vi "Set UI Busy State.vi"(7 "Defer Panel Updates":bool, 8 "error in (no error)":errorcluster, 11 "VI in":refnum<vi>) -> (0 "error out":errorcluster, 3 "VI out":refnum<vi>)   [LabVIEW 2019, in "DSF Core.lvlib"]
uses:
  DSF Core.lvlib
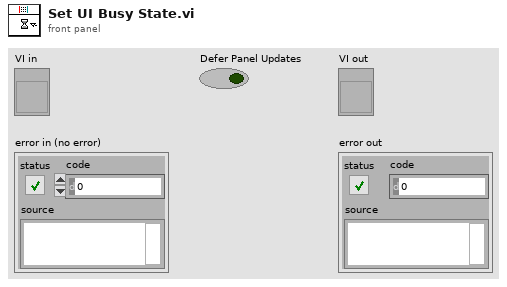
[diagram p1: front panel]
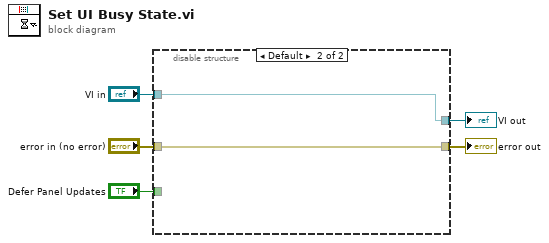
[diagram p0: block diagram]
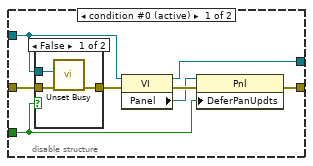
[diagram p2: hidden frame]
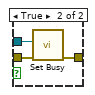
[diagram p3: hidden frame]
diagram:
  n1 = disable-structure shown="Default" {
    disable-tunnel: [w13 w20] -> w5
    disable-tunnel: [w11 w21] -> w4
    disable-tunnel: "VI in" -> [w9 w21]
    disable-tunnel: "error in (no error)" -> [w8 w20]
    disable-tunnel: "Defer Panel Updates" -> [w6 _]
    frame condition #0 (active) {
      n2 = case shown="False" w6 {
        tunnel: w9 -> [w16 w19]
        tunnel: w8 -> [w15 w18]
        tunnel: [w14 w17] -> w7
        frame False {
          n3 = call <vilib>:"Unset Busy.vi"("error in (no error)"=w15, "VI reference (current VI)"=w16) -> ("error out"=w14:errorcluster)  [unwired: 9 in]
        }
        frame True {
          n4 = call <vilib>:"Set Busy.vi"("error in (no error)"=w18, "VI reference (current VI)"=w19) -> ("error out"=w17:errorcluster)  [unwired: 8 in, 1 out]
        }
      }
      n5 = property class="VI"(reference=w9, error in=w7) -> (reference out=w11:refnum<vi>, error out=w12:errorcluster, "Panel"=w10:refnum<vi>)
      n6 = property class="Pnl"(reference=w10, error in=w12, "DeferPanUpdts"=w6) -> (error out=w13:errorcluster)  [unwired: 1 out]
    }
    frame condition #1 {
    }
  }
  "error out" <- w5
  "VI out" <- w4
